vi "ReplaceInMatrice19x19.vi"(11 "Input Array":dbl[](array[numeric])) -> (0 "Output Array":dbl[][](array[numeric]))   [LabVIEW 2022 SP3]
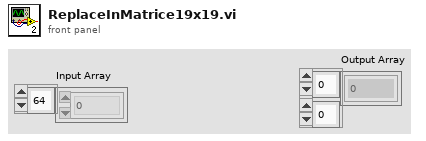
[diagram p1: front panel]
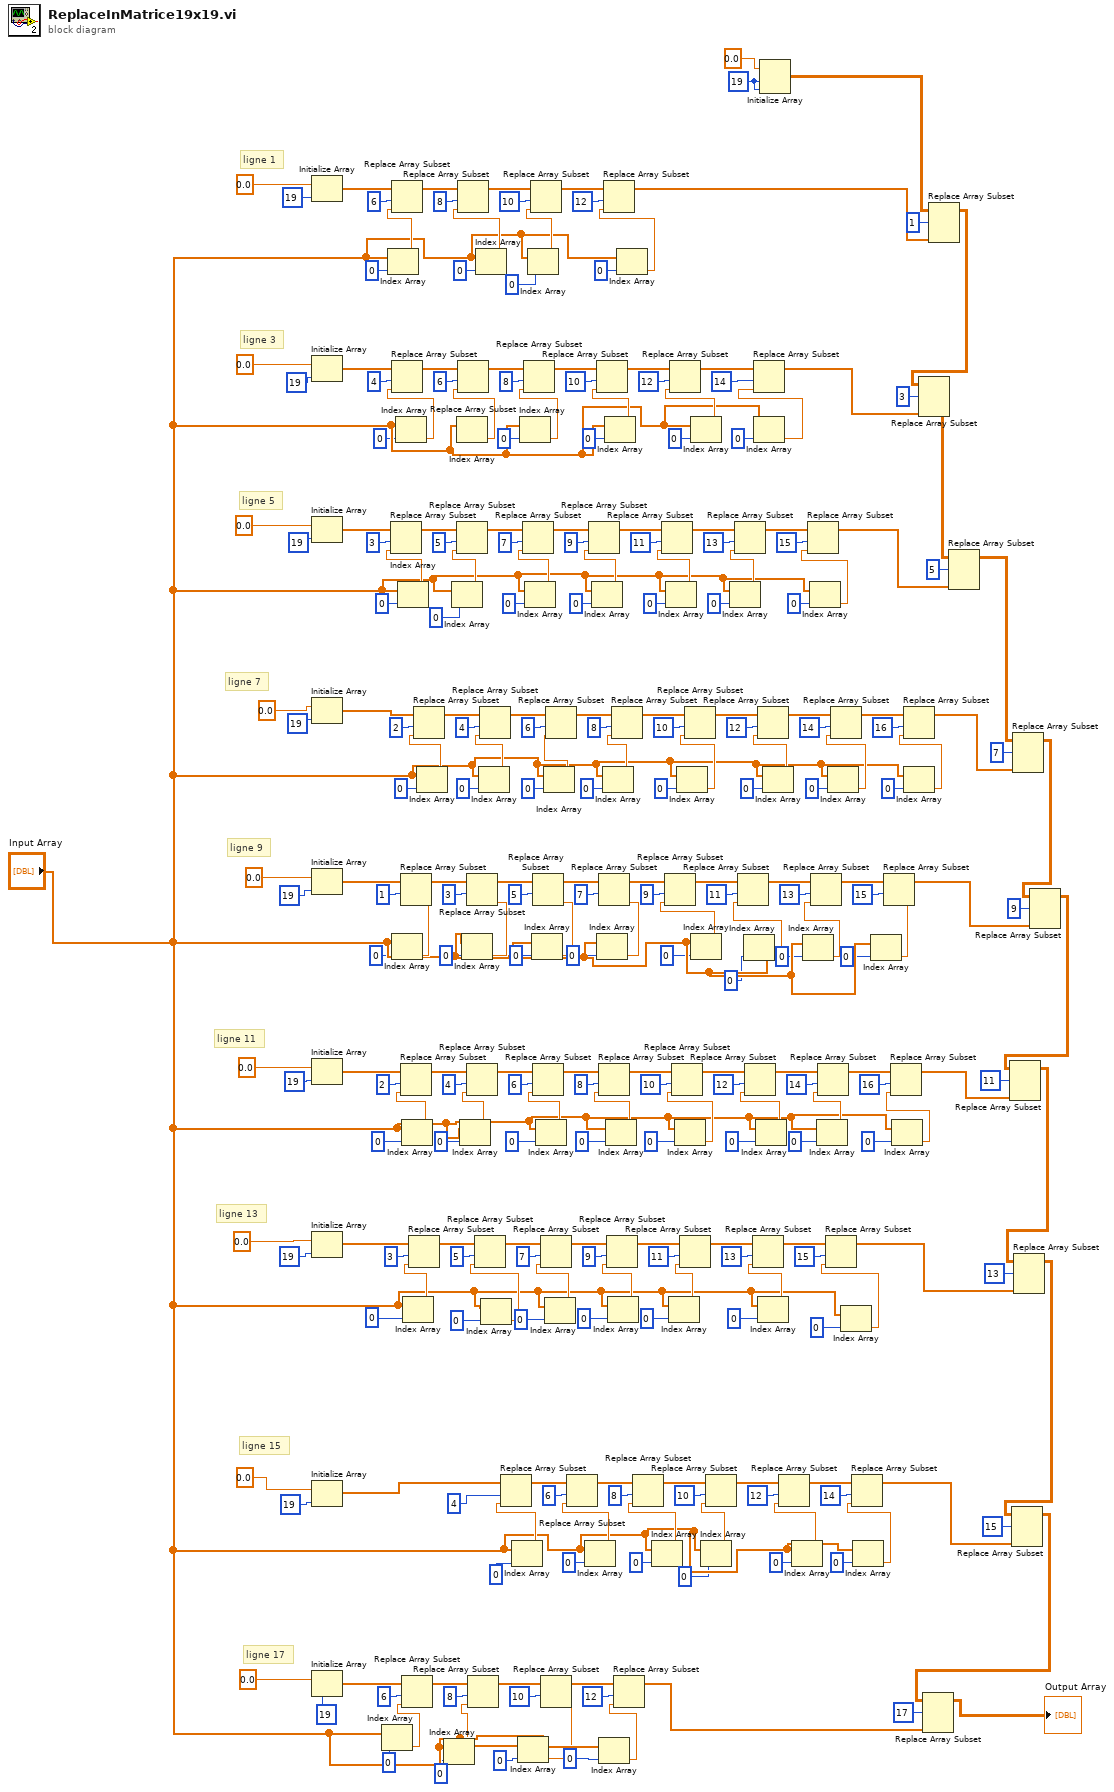
[diagram p0: block diagram]
diagram:
  w279 = 19
  # "ligne 17"
  # "ligne 15"
  # "ligne 13"
  # "ligne 11"
  # "ligne 9"
  # "ligne 7"
  # "ligne 5"
  # "ligne 3"
  # "ligne 1"
  n1 = Initialize Array(0.0 ("element"), 19 ("dimension size")) -> (w276:dbl[])
  n2 = Initialize Array(0.0 ("element"), 19 ("dimension size")) -> (w256:dbl[])
  n3 = Initialize Array(0.0 ("element"), 19 ("dimension size")) -> (w242:dbl[])
  n4 = Initialize Array(0.0 ("element"), 19 ("dimension size")) -> (w224:dbl[])
  n5 = Initialize Array(0.0 ("element"), 19 ("dimension size")) -> (w205:dbl[])
  n6 = Initialize Array(0.0 ("element"), 19 ("dimension size")) -> (w188:dbl[])
  n7 = Initialize Array(0.0 ("element"), 19 ("dimension size")) -> (w172:dbl[])
  n8 = Initialize Array(0.0 ("element"), 19 ("dimension size")) -> (w156:dbl[])
  n9 = Initialize Array(0.0 ("element"), 19 ("dimension size")) -> (w152:dbl[])
  n10 = Index Array(array="Input Array", index=0) -> (element=w86:dbl)
  n11 = Index Array(array="Input Array", index=0) -> (element=w133:dbl)
  n12 = Replace Array Subset(array=w276, new element=w133, index=6) -> (w275:dbl[])
  n13 = Index Array(array="Input Array", index=0) -> (element=w144:dbl)
  n14 = Index Array(array="Input Array", index=0) -> (element=w132:dbl)
  n15 = Replace Array Subset(array=w256, new element=w132, index=4) -> (w257:dbl[])
  n16 = Index Array(array="Input Array", index=0) -> (element=w126:dbl)
  n17 = Replace Array Subset(array=w242, new element=w126, index=3) -> (w243:dbl[])
  n18 = Replace Array Subset(array=w205, new element=w144, index=1) -> (w204:dbl[])
  n19 = Index Array(array="Input Array", index=0) -> (element=w104:dbl)
  n20 = Replace Array Subset(array=w188, new element=w104, index=2) -> (w189:dbl[])
  n21 = Replace Array Subset(array=w152, new element=w86, index=6) -> (w151:dbl[])
  n22 = Index Array(array="Input Array", index=0) -> (element=w103:dbl)
  n23 = Replace Array Subset(array=w172, new element=w103, index=3) -> (w173:dbl[])
  n24 = Index Array(array="Input Array", index=0) -> (element=w119:dbl)
  n25 = Replace Array Subset(array=w224, new element=w119, index=2) -> (w225:dbl[])
  n26 = Index Array(array="Input Array", index=0) -> (element=w87:dbl)
  n27 = Index Array(array="Input Array", index=0) -> (element=w125:dbl)
  n28 = Index Array(array="Input Array") -> (element=w131:dbl)  [unwired: 1 in]
  n29 = Replace Array Subset(array=w243, new element=w125, index=5) -> (w252:dbl[])
  n30 = Replace Array Subset(array=w257, new element=w131, index=6) -> (w266:dbl[])
  n31 = Index Array(array="Input Array", index=0) -> (element=w105:dbl)
  n32 = Index Array(array="Input Array", index=0) -> (element=w143:dbl)
  n33 = Replace Array Subset(array=w204, new element=w143, index=3) -> (w209:dbl[])
  n34 = Replace Array Subset(array=w189, new element=w105, index=4) -> (w191:dbl[])
  n35 = Replace Array Subset(array=w151, new element=w87, index=8) -> (w150:dbl[])
  n36 = Index Array(array="Input Array", index=0) -> (element=w134:dbl)
  n37 = Replace Array Subset(array=w275, new element=w134, index=8) -> (w274:dbl[])
  n38 = Index Array(array="Input Array", index=0) -> (element=w118:dbl)
  n39 = Replace Array Subset(array=w225, new element=w118, index=4) -> (w227:dbl[])
  n40 = Index Array(array="Input Array", index=0) -> (element=w102:dbl)
  n41 = Replace Array Subset(array=w173, new element=w102, index=5) -> (w182:dbl[])
  n42 = Index Array(array="Input Array", index=0) -> (element=w91:dbl)
  n43 = Replace Array Subset(array=w156, new element=w91, index=4) -> (w157:dbl[])
  n44 = Index Array(array="Input Array", index=0) -> (element=w88:dbl)
  n45 = Index Array(array="Input Array", index=0) -> (element=w127:dbl)
  n46 = Replace Array Subset(array=w266, new element=w127, index=8) -> (w265:dbl[])
  n47 = Index Array(array="Input Array", index=0) -> (element=w124:dbl)
  n48 = Replace Array Subset(array=w252, new element=w124, index=7) -> (w251:dbl[])
  n49 = Index Array(array="Input Array", index=0) -> (element=w135:dbl)
  n50 = Replace Array Subset(array=w274, new element=w135, index=10) -> (w273:dbl[])
  n51 = Index Array(array="Input Array", index=0) -> (element=w142:dbl)
  n52 = Replace Array Subset(array=w209, new element=w142, index=5) -> (w218:dbl[])
  n53 = Index Array(array="Input Array", index=0) -> (element=w106:dbl)
  n54 = Replace Array Subset(array=w191, new element=w106, index=6) -> (w200:dbl[])
  n55 = Replace Array Subset(array=w150, new element=w88, index=10) -> (w149:dbl[])
  n56 = Index Array(array="Input Array", index=0) -> (element=w117:dbl)
  n57 = Index Array(array="Input Array", index=0) -> (element=w101:dbl)
  n58 = Replace Array Subset(array=w182, new element=w101, index=7) -> (w181:dbl[])
  n59 = Replace Array Subset(array=w227, new element=w117, index=6) -> (w236:dbl[])
  n60 = Index Array(array="Input Array", index=0) -> (element=w92:dbl)
  n61 = Replace Array Subset(array=w157, new element=w92, index=6) -> (w166:dbl[])
  n62 = Index Array(array="Input Array", index=0) -> (element=w123:dbl)
  n63 = Replace Array Subset(array=w251, new element=w123, index=9) -> (w250:dbl[])
  n64 = Index Array(array="Input Array", index=0) -> (element=w141:dbl)
  n65 = Replace Array Subset(array=w218, new element=w141, index=7) -> (w217:dbl[])
  n66 = Index Array(array="Input Array", index=0) -> (element=w89:dbl)
  n67 = Index Array(array="Input Array", index=0) -> (element=w116:dbl)
  n68 = Index Array(array="Input Array", index=0) -> (element=w128:dbl)
  n69 = Replace Array Subset(array=w265, new element=w128, index=10) -> (w264:dbl[])
  n70 = Index Array(array="Input Array", index=0) -> (element=w107:dbl)
  n71 = Replace Array Subset(array=w200, new element=w107, index=8) -> (w199:dbl[])
  n72 = Index Array(array="Input Array", index=0) -> (element=w100:dbl)
  n73 = Replace Array Subset(array=w181, new element=w100, index=9) -> (w180:dbl[])
  n74 = Replace Array Subset(array=w236, new element=w116, index=8) -> (w235:dbl[])
  n75 = Replace Array Subset(array=w149, new element=w89, index=12) -> (w10:dbl[])
  n76 = Index Array(array="Input Array", index=0) -> (element=w136:dbl)
  n77 = Replace Array Subset(array=w273, new element=w136, index=12) -> (w27:dbl[])
  n78 = Index Array(array="Input Array", index=0) -> (element=w93:dbl)
  n79 = Replace Array Subset(array=w166, new element=w93, index=8) -> (w165:dbl[])
  n80 = Index Array(array="Input Array", index=0) -> (element=w122:dbl)
  n81 = Replace Array Subset(array=w250, new element=w122, index=11) -> (w245:dbl[])
  n82 = Index Array(array="Input Array", index=0) -> (element=w99:dbl)
  n83 = Index Array(array="Input Array", index=0) -> (element=w108:dbl)
  n84 = Replace Array Subset(array=w199, new element=w108, index=10) -> (w198:dbl[])
  n85 = Index Array(array="Input Array", index=0) -> (element=w115:dbl)
  n86 = Replace Array Subset(array=w180, new element=w99, index=11) -> (w175:dbl[])
  n87 = Replace Array Subset(array=w235, new element=w115, index=10) -> (w234:dbl[])
  n88 = Index Array(array="Input Array", index=0) -> (element=w129:dbl)
  n89 = Replace Array Subset(array=w264, new element=w129, index=12) -> (w259:dbl[])
  n90 = Index Array(array="Input Array", index=0) -> (element=w140:dbl)
  n91 = Replace Array Subset(array=w217, new element=w140, index=9) -> (w216:dbl[])
  n92 = Index Array(array="Input Array", index=0) -> (element=w94:dbl)
  n93 = Replace Array Subset(array=w165, new element=w94, index=10) -> (w164:dbl[])
  n94 = Index Array(array="Input Array", index=0) -> (element=w121:dbl)
  n95 = Replace Array Subset(array=w245, new element=w121, index=13) -> (w240:dbl[])
  n96 = Index Array(array="Input Array", index=0) -> (element=w139:dbl)
  n97 = Replace Array Subset(array=w216, new element=w139, index=11) -> (w211:dbl[])
  n98 = Index Array(array="Input Array", index=0) -> (element=w130:dbl)
  n99 = Replace Array Subset(array=w259, new element=w130, index=14) -> (w17:dbl[])
  n100 = Index Array(array="Input Array", index=0) -> (element=w109:dbl)
  n101 = Replace Array Subset(array=w198, new element=w109, index=12) -> (w193:dbl[])
  n102 = Index Array(array="Input Array", index=0) -> (element=w98:dbl)
  n103 = Replace Array Subset(array=w175, new element=w98, index=13) -> (w170:dbl[])
  n104 = Initialize Array(0.0, w279, w279) -> (w28:dbl[][])
  n105 = Index Array(array="Input Array", index=0) -> (element=w114:dbl)
  n106 = Replace Array Subset(array=w234, new element=w114, index=12) -> (w229:dbl[])
  n107 = Index Array(array="Input Array", index=0) -> (element=w95:dbl)
  n108 = Replace Array Subset(array=w164, new element=w95, index=12) -> (w159:dbl[])
  n109 = Index Array(array="Input Array", index=0) -> (element=w138:dbl)
  n110 = Index Array(array="Input Array", index=0) -> (element=w120:dbl)
  n111 = Replace Array Subset(array=w240, new element=w120, index=15) -> (w16:dbl[])
  n112 = Replace Array Subset(array=w211, new element=w138, index=13) -> (w207:dbl[])
  n113 = Index Array(array="Input Array", index=0) -> (element=w110:dbl)
  n114 = Replace Array Subset(array=w193, new element=w110, index=14) -> (w186:dbl[])
  n115 = Index Array(array="Input Array", index=0) -> (element=w113:dbl)
  n116 = Replace Array Subset(array=w229, new element=w113, index=14) -> (w222:dbl[])
  n117 = Index Array(array="Input Array", index=0) -> (element=w97:dbl)
  n118 = Replace Array Subset(array=w170, new element=w97, index=15) -> (w12:dbl[])
  n119 = Index Array(array="Input Array", index=0) -> (element=w96:dbl)
  n120 = Replace Array Subset(array=w159, new element=w96, index=14) -> (w11:dbl[])
  n121 = Index Array(array="Input Array", index=0) -> (element=w137:dbl)
  n122 = Replace Array Subset(array=w207, new element=w137, index=15) -> (w14:dbl[])
  n123 = Index Array(array="Input Array", index=0) -> (element=w111:dbl)
  n124 = Replace Array Subset(array=w186, new element=w111, index=16) -> (w13:dbl[])
  n125 = Index Array(array="Input Array", index=0) -> (element=w112:dbl)
  n126 = Replace Array Subset(array=w222, new element=w112, index=16) -> (w15:dbl[])
  n127 = Replace Array Subset(array=w28, new element=w27, index (row)=1) -> (w25:dbl[][])  [unwired: 1 in]
  n128 = Replace Array Subset(array=w25, new element=w17, index (row)=3) -> (w24:dbl[][])  [unwired: 1 in]
  n129 = Replace Array Subset(array=w24, new element=w16, index (row)=5) -> (w23:dbl[][])  [unwired: 1 in]
  n130 = Replace Array Subset(array=w23, new element=w15, index (row)=7) -> (w22:dbl[][])  [unwired: 1 in]
  n131 = Replace Array Subset(array=w22, new element=w14, index (row)=9) -> (w21:dbl[][])  [unwired: 1 in]
  n132 = Replace Array Subset(array=w21, new element=w13, index (row)=11) -> (w20:dbl[][])  [unwired: 1 in]
  n133 = Replace Array Subset(array=w20, new element=w12, index (row)=13) -> (w19:dbl[][])  [unwired: 1 in]
  n134 = Replace Array Subset(array=w19, new element=w11, index (row)=15) -> (w18:dbl[][])  [unwired: 1 in]
  n135 = Replace Array Subset(array=w18, new element=w10, index (row)=17) -> (→"Output Array":dbl[][])  [unwired: 1 in]
